vi "Unregister AEs.vi"(8 "error in (no error)":errorcluster, 10 "Unregister Info":T1, 11 "CS++PVMonitor in":refnum<class "CS++PVMonitor.lvclass">) -> (0 "error out":errorcluster, 3 "CS++PVMonitor out":refnum<class "CS++PVMonitor.lvclass">)   [LabVIEW 2015, in "CS++PVMonitor.lvlib" / "CS++PVMonitor.lvclass"]
doc: "Unregister alarm and event monitoring for process variables."
uses:
  CS++PVMonitor.lvclass
  <vilib>/ActorFramework/Message Enqueuer/Message Enqueuer.lvclass
  CS++PVMonitor.lvclass/CS++PVMonitor.ctl
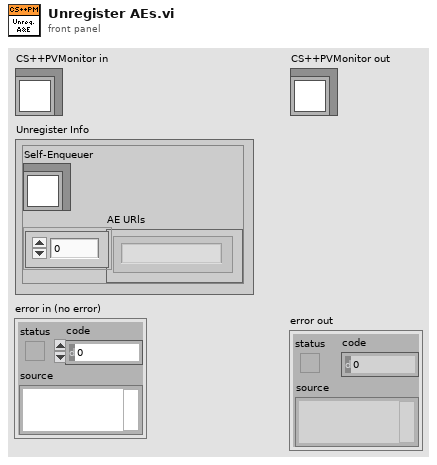
[diagram p1: front panel]
types:
  T1 = cluster{"Self-Enqueuer":refnum<class "Message Enqueuer.lvclass">, "AE URls":string[]}
  T2 = cluster{"PV URL":string, "Observers":cluster{"Enqueuer":refnum<class "Message Enqueuer.lvclass">, "CS++AEUpdate Msg":refnum<class "CS++AEUpdate Msg.lvclass">}[]}[]
  T3 = cluster{"PV URL":string, "Observers":cluster{"Enqueuer":refnum<class "Message Enqueuer.lvclass">, "CS++AEUpdate Msg":refnum<class "CS++AEUpdate Msg.lvclass">}[]}
  T4 = cluster{"Enqueuer":refnum<class "Message Enqueuer.lvclass">, "CS++AEUpdate Msg":refnum<class "CS++AEUpdate Msg.lvclass">}[]
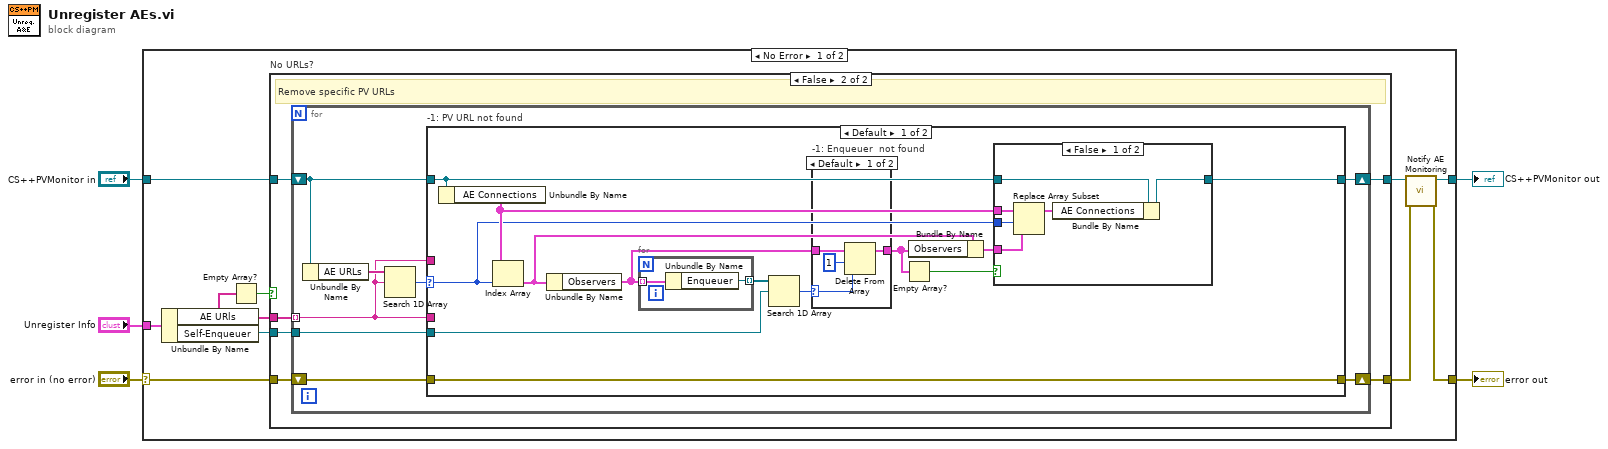
[diagram p0: block diagram]
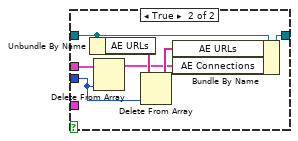
[diagram p3: hidden frame]
diagram:
  n1 = case shown="No Error" "error in (no error)" {
    selector: "error in (no error)" -> [w14 w68]
    tunnel: [w9 w68] -> w1
    tunnel: [w10 w67] -> w2
    tunnel: "CS++PVMonitor in" -> [w13 w67]
    tunnel: "Unregister Info" -> [w15 _]
    frame No Error {
      n2 = Unbundle By Name(w15) -> ("AE URls"=w7:string[], "Self-Enqueuer"=w12:refnum<class "Message Enqueuer.lvclass">)
      n3 = Empty Array?(array=w7) -> (empty?=w6:bool)
      n4 = case "No URLs?" shown="False" w6 {
        tunnel: w7 -> [_ w23]
        tunnel: w14 -> [w16 w22]
        tunnel: [w16 w21] -> w8
        tunnel: w13 -> [w17 w20]
        tunnel: [w17 w19] -> w11
        tunnel: w12 -> [_ w18]
        frame True {
          # "Remove observer from all PV URLs; to be implemented!"
        }
        frame False {
          # "Remove specific PV URLs"
          n5 = for {
            tunnel: w23 -> [w24] mode=indexing
            shift-right: [w26] -> w21
            shift-left: w22 -> [w25]
            shift-right: [w27] -> w19
            shift-left: w20 -> [w29]
            tunnel: w18 -> [w28]
            n6 = Unbundle By Name(w29) -> ("AE URLs"=w31:string[])
            n7 = Search 1D Array(1D array=w31, element=w24) -> (index of element=w30:i32)  [unwired: 1 in]
            n8 = case "-1: PV URL not found" shown="Default" w30 {
              selector: w30 -> [w41 _]
              tunnel: w29 -> [w36 w66]
              tunnel: w28 -> [w39 _]
              tunnel: w24 -> [_ _]
              tunnel: [w34 w66] -> w27
              tunnel: [w35 w65] -> w26
              tunnel: w25 -> [w35 w65]
              tunnel: w24 -> [_ _]
              frame Default {
                n9 = Unbundle By Name(w36) -> ("AE Connections"=w42:T2)
                n10 = Index Array(array=w42, index=w41) -> (element=w40:T3)
                n11 = Unbundle By Name(w40) -> ("Observers"=w43:T4)
                n12 = for {
                  tunnel: w43 -> [w64] mode=indexing
                  tunnel: [w63] -> w44 mode=indexing
                  n13 = Unbundle By Name(w64) -> ("Enqueuer"=w63:refnum<class "Message Enqueuer.lvclass">)
                }
                n14 = Search 1D Array(1D array=w44, element=w39) -> (index of element=w37:i32)  [unwired: 1 in]
                n15 = case "-1: Enqueuer  not found" shown="Default" w37 {
                  selector: w37 -> [w59 _]
                  tunnel: w43 -> [w61 w62]
                  tunnel: [w60 w62] -> w32
                  frame Default {
                    n16 = Delete From Array(array=w61, length=1, index=w59) -> (array with subset deleted=w60:T4)  [unwired: 1 out]
                  }
                  frame -1 {
                  }
                }
                n17 = Empty Array?(array=w32) -> (empty?=w33:bool)
                n18 = Bundle By Name(cluster=w40, "Observers"=w32) -> (w38:T3)
                n19 = case shown="False" w33 {
                  tunnel: w42 -> [w50 w57]
                  tunnel: w41 -> [w49 w55]
                  tunnel: w38 -> [w48 _]
                  tunnel: w36 -> [w47 w54]
                  tunnel: [w46 w52] -> w34
                  frame False {
                    n20 = Replace Array Subset(array=w50, new element=w48, index=w49) -> (w45:T2)
                    n21 = Bundle By Name(cluster=w47, "AE Connections"=w45) -> (w46:refnum<class "CS++PVMonitor.lvclass">)
                  }
                  frame True {
                    n22 = Unbundle By Name(w54) -> ("AE URLs"=w56:string[])
                    n23 = Delete From Array(array=w57, index=w55) -> (array with subset deleted=w51:T2)  [unwired: 1 in, 1 out]
                    n24 = Delete From Array(array=w56, index=w55) -> (array with subset deleted=w53:string[])  [unwired: 1 in, 1 out]
                    n25 = Bundle By Name(cluster=w54, "AE URLs"=w53, "AE Connections"=w51) -> (w52:refnum<class "CS++PVMonitor.lvclass">)
                  }
                }
              }
              frame -1 {
              }
            }
          }
        }
      }
      n26 = call-dynamic "Notify AE Monitoring.vi"("error in (no error)"=w8, "CS++PVMonitor in"=w11) -> ("error out"=w9:errorcluster, "CS++PVMonitor out"=w10:refnum<class "CS++PVMonitor.lvclass">)  [unwired: 8 in]
    }
    frame Error {
    }
  }
  "error out" <- w1
  "CS++PVMonitor out" <- w2
